vi "SetTWPos.vi"(8 "error in (no error)":errorcluster, 10 "Tick Pos":dbl) -> (0 "error out":errorcluster)   [LabVIEW 2015]
uses:
  TW Global.vi
panel:
  out "Set Rotation":dbl
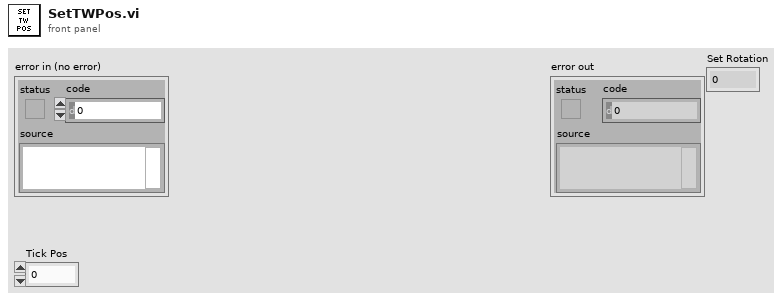
[diagram p1: front panel]
types:
  T1 = typedef "PortC Settings Type Def.ctl" = cluster{"Down":dbl, "Up":dbl, "Increments":dbl}
  T2 = typedef "Detailed Motor Type Def.ctl" = cluster{"MotorRef":T3, "Encoder Ticks Per Rev":dbl, "Set Position":dbl, "Wheel Radius":dbl}
  T3 = typedef "WPI_MotorControlDeviceRef.ctl" = cluster{"DeviceStatus":errorcluster, "Type":T4, "PWM":cluster{"PWM Channel":T5, "DeadBand":T6}, "CAN":cluster{"Device Number":u8, "Control Mode":T7, "Semaphore":T8, "Max Vout":dbl, "TalonSRX Control Mode":T9}, "Invert":bool}
  T4 = typedef "WPI_MotorControlType.ctl" = enum16{"PWM", "CAN", "CANTalonSRX"}
  T5 = typedef "FPGA_DIOPWMChannel.ctl" = enum8{"PWM 0", "PWM 1", "PWM 2", "PWM 3", "PWM 4", "PWM 5", "PWM 6", "PWM 7", "PWM 8", "PWM 9", "PWM MXP 0", "PWM MXP 1", "PWM MXP 2", "PWM MXP 3", "PWM MXP 4", "PWM MXP 5", "PWM MXP 6", "PWM MXP 7", "PWM MXP 8", "PWM MXP 9", "Invalid"}
  T6 = typedef "WPI_PWMDeadband.ctl" = cluster{"Name":string, "maxPositivePwm":i32, "minPositivePwm":i32, "centerPwm":i32, "maxNegativePwm":i32, "minNegativePwm":i32, "angularRange":u16}
  T7 = typedef "WPI_CANJaguar_ControlMode.ctl" = enum8{"Percent VBus", "Current", "Speed", "Position", "Voltage"}
  T8 = typedef "Semaphore RefNum" = refnum<k1>
  T9 = typedef "WPI_CANTalonSRX_APIControlMode.ctl" = enum8{"Percent VBus", "Speed", "Position", "Slave", "Unchanged / Invalid", "Voltage Compensation", "Current", "Motion Profile"}
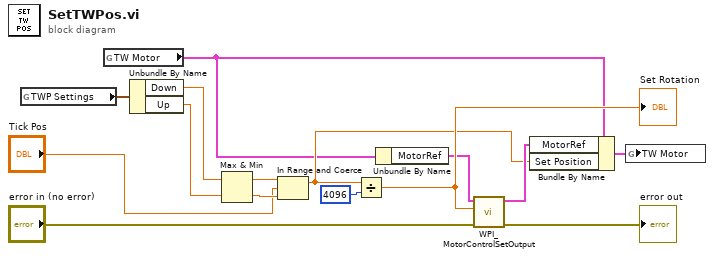
[diagram p0: block diagram]
diagram:
  n1 = global read "TW Global.vi" "TWP Settings"() -> (w7:T1)
  n2 = global read "TW Global.vi" "TW Motor"() -> (w2:T2)
  n3 = Unbundle By Name(w7) -> ("Down"=w9:dbl, "Up"=w8:dbl)
  n4 = Max & Min(x=w9, y=w8) -> (max(x,y)=w5:dbl, min(x,y)=w6:dbl)
  n5 = In Range and Coerce(upper limit=w5, x="Tick Pos", lower limit=w6) -> (coerced(x)=w10:dbl)  [unwired: 1 out]
  n6 = Divide(x=w10, y=4096) -> (x/y=w15:dbl)
  "Set Rotation" <- w15
  n7 = Unbundle By Name(w2) -> ("MotorRef"=w14:T3)
  n8 = call <vilib>:"WPI_MotorControlSetOutput.vi"("error in (no error)"="error in (no error)", "Output"=w15, "MotorControlDevRef"=w14) -> ("error out"=→"error out":errorcluster, "MotorControlDevRef"=w11:T3)  [unwired: 6 in, 1 out]
  n9 = Bundle By Name(cluster=w2, "MotorRef"=w11, "Set Position"=w10) -> (w1:T2)
  n10 = global write "TW Global.vi" "TW Motor"(w1) -> ()
